vi "MAINP Update Ports.vi"(7 "Controls":refnum<vi>[](array[refnum]), 8 "error in (no error)":errorcluster, 11 "Device Item Ref in":T1 format="%.0x") -> (0 "error out":errorcluster, 3 "Device Item Ref out":T1 format="%.0x")   [LabVIEW 2018, in "CAN Gateway System Explorer.lvlib"]
uses:
  CAN Gateway System Explorer.lvlib
  <vilib>/NI Veristand/Custom Device API/Custom Device Item Ref.ctl
  Shared/Constants.vi
  <vilib>/NI Veristand/Custom Device API/Get Item Property (String).vi
  <vilib>/NI Veristand/Custom Device API/Custom Device API.lvlib
  Shared/CAN Gateway Shared.lvlib
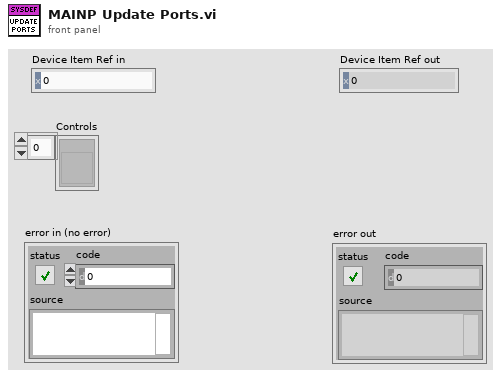
[diagram p1: front panel]
types:
  T1 = typedef "Custom Device API.lvlib/Custom Device Item Ref.ctl" = u64
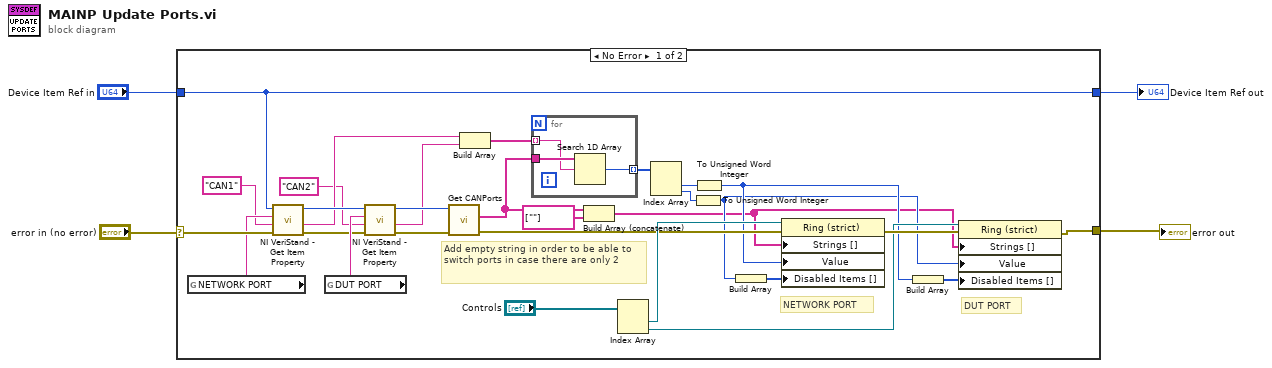
[diagram p0: block diagram]
diagram:
  n1 = case shown="No Error" "error in (no error)" {
    selector: "error in (no error)" -> [w33 w38]
    tunnel: "Device Item Ref in" -> [w23 w37]
    tunnel: [w23 w37] -> w2
    tunnel: [w17 w38] -> w1
    frame No Error {
      # "Add empty string in order to be able to switch ports in case there are only 2"
      # "DUT PORT"
      # "NETWORK PORT"
      n2 = global read "Constants.vi" "NETWORK PORT"() -> (w32:string)
      n3 = call-poly <vilib>:"NI VeriStand - Get Item Property.vi"("error in (no error)"=w33, "Default Value"="CAN1", "Property Name"=w32, "Item Ref in"=w23) -> ("error out"=w29:errorcluster, "Value"=w26:string, "Item Ref out"=w31:T1)  [unwired: 4 in, 1 out]
      n4 = global read "Constants.vi" "DUT PORT"() -> (w30:string)
      n5 = call-poly <vilib>:"NI VeriStand - Get Item Property.vi"("error in (no error)"=w29, "Default Value"="CAN2", "Property Name"=w30, "Item Ref in"=w31) -> ("error out"=w27:errorcluster, "Value"=w25:string, "Item Ref out"=w28:T1)  [unwired: 4 in, 1 out]
      n6 = call "Get CANPorts.vi"("error in (no error)"=w27, "Device Item Ref in"=w28) -> ("error out"=w20:errorcluster, "CAN Ports"=w9:string[])  [unwired: 7 in, 1 out]
      n7 = Build Array(w26, w25) -> (w24:string[])
      n8 = for {
        tunnel: w24 -> [w35] mode=indexing
        tunnel: w9 -> [w36]
        tunnel: [w34] -> w19 mode=indexing
        n9 = Search 1D Array(1D array=w36, element=w35) -> (index of element=w34:i32)  [unwired: 1 in]
      }
      n10 = Build Array (concatenate)(w9, string[] [""] ("element")) -> (w7:string[])
      n11 = Index Array(array="Controls") -> (element #1=w21:refnum<vi>, element #2=w16:refnum<vi>)  [unwired: 2 in]
      n12 = Index Array(array=w19) -> (element #1=w15:i32, element #2=w14:i32)  [unwired: 2 in]
      n13 = To Unsigned Word Integer(number=w14) -> (unsigned 16bit integer=w10:u16)
      n14 = To Unsigned Word Integer(number=w15) -> (unsigned 16bit integer=w12:u16)
      n15 = Build Array(w10) -> (w13:u16[])
      n16 = property class="Ring (strict)"(reference=w21, error in=w20, "Strings []"=w7, "Value"=w12, "Disabled Items []"=w13) -> (error out=w18:errorcluster)  [unwired: 1 out]
      n17 = Build Array(w12) -> (w11:u16[])
      n18 = property class="Ring (strict)"(reference=w16, error in=w18, "Strings []"=w7, "Value"=w10, "Disabled Items []"=w11) -> (error out=w17:errorcluster)  [unwired: 1 out]
    }
    frame Error {
    }
  }
  "error out" <- w1
  "Device Item Ref out" <- w2
